vi "get_status.vi"(0 "connection ID in":refnum<k5>, 2 "command in":string, 3 "error in":errorcluster, 4 "设备编号":u8) -> (5 "connection ID out":refnum<k5>, 6 "Status received":string[](array[string]), 7 "error out":errorcluster)   [LabVIEW 2013]
panel:
  out "bytes written":i32
  out "Data Length":u16
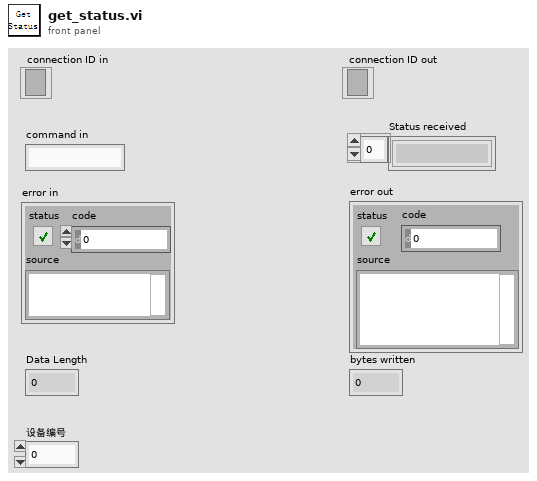
[diagram p1: front panel]
types:
  T1 = enum16{"Standard", "Buffered", "CRLF", "Immediate"}
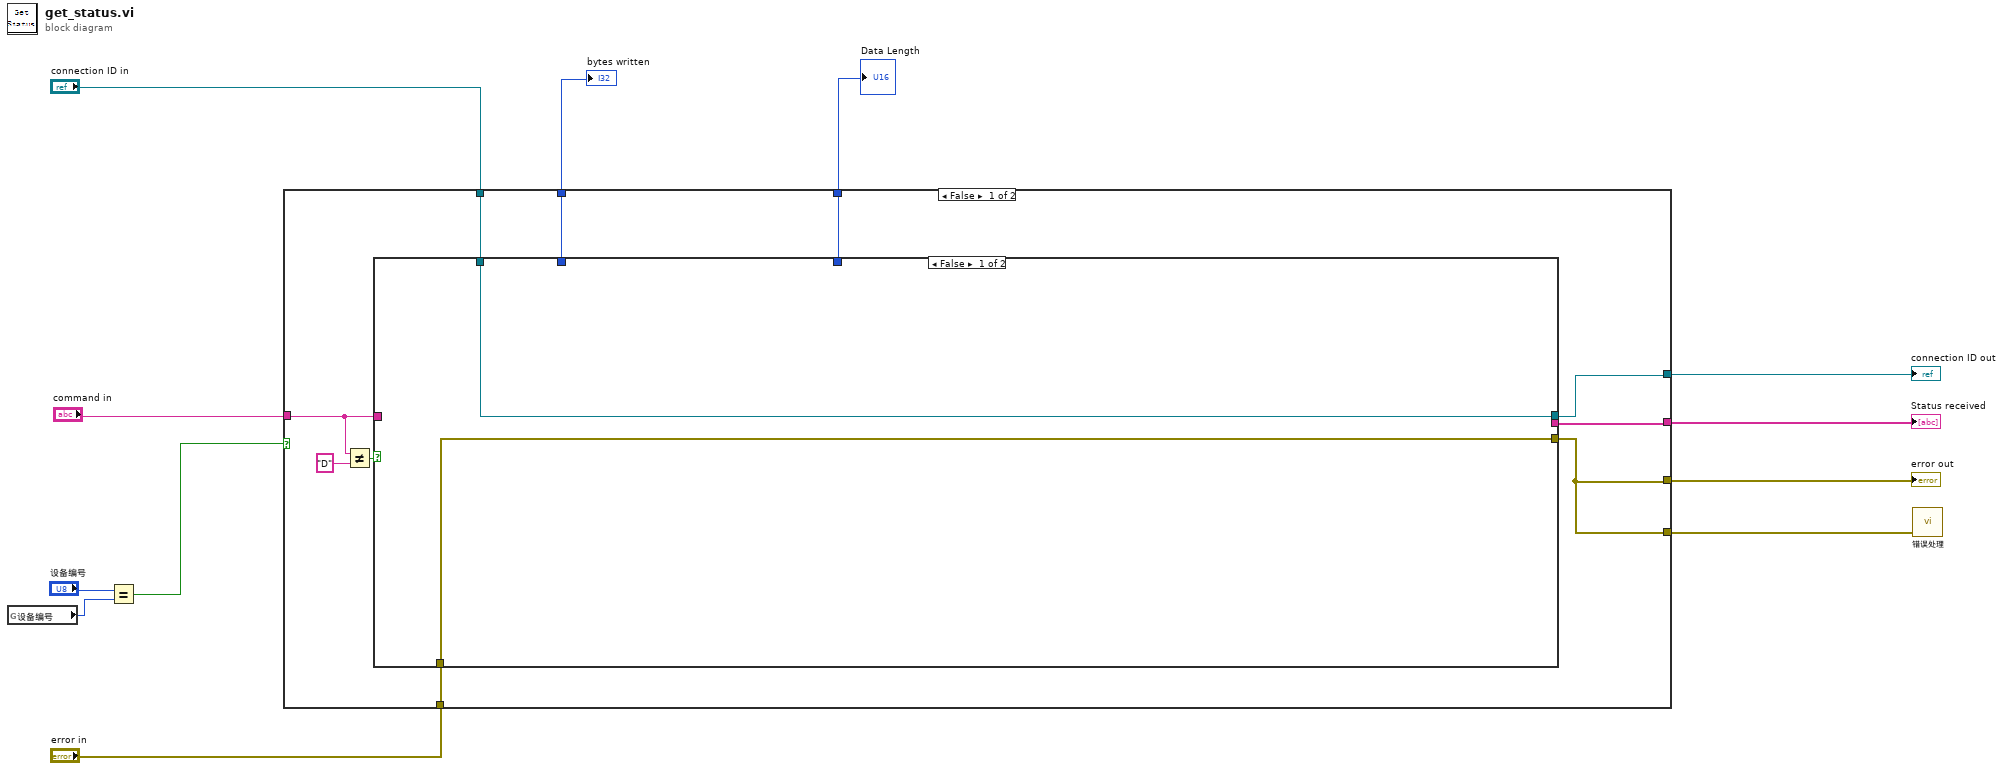
[diagram p0: block diagram]
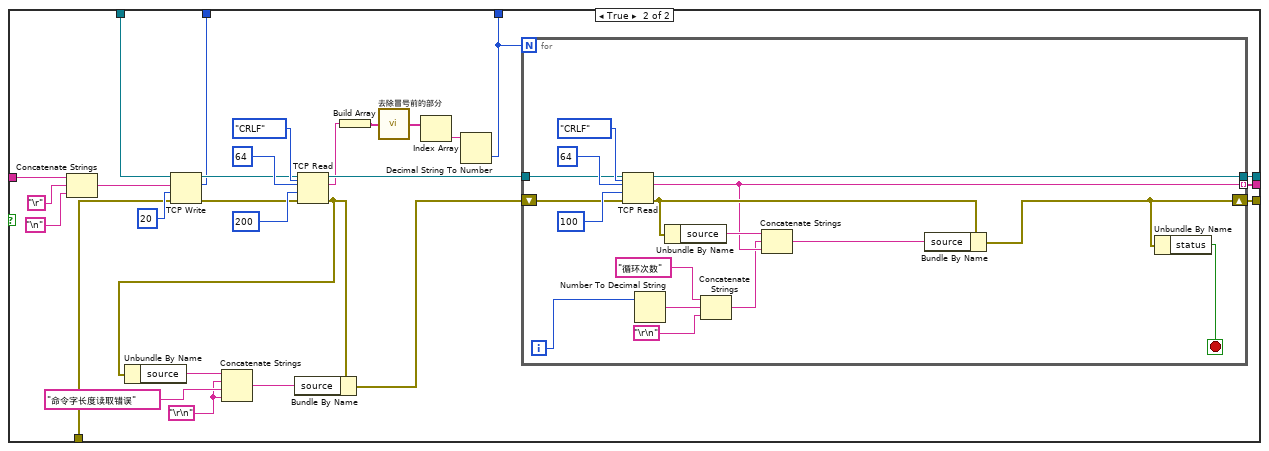
[diagram p2: hidden frame]
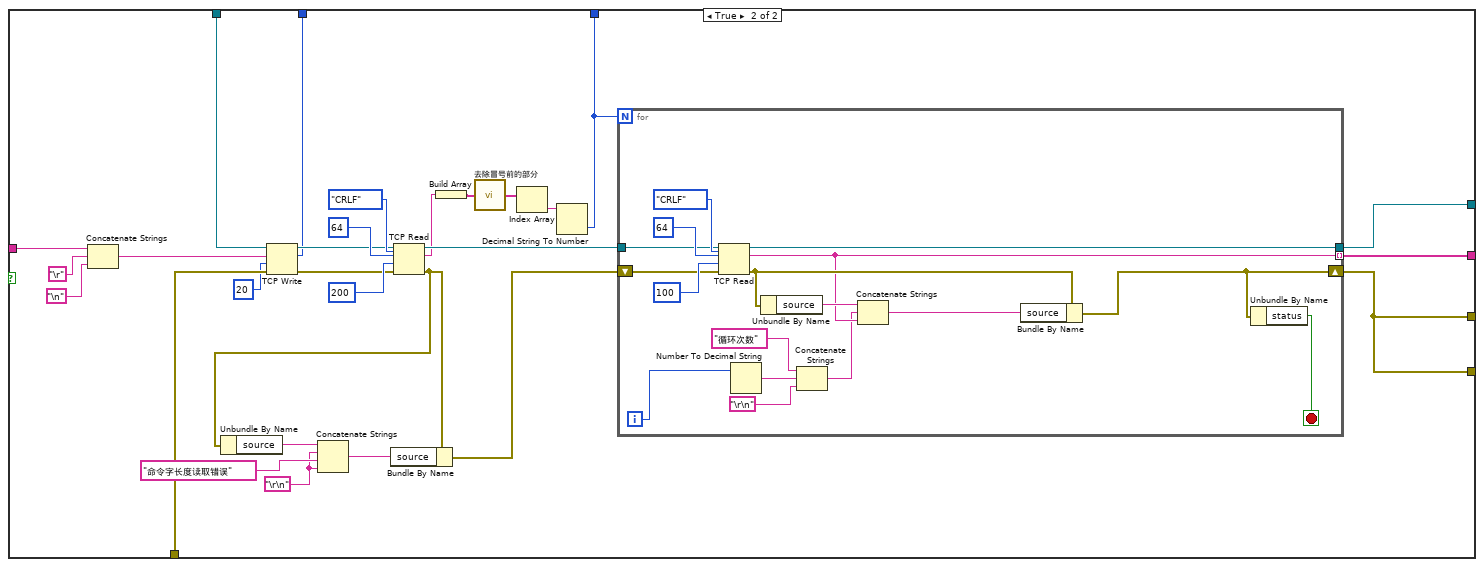
[diagram p3: hidden frame]
diagram:
  n1 = global read "设备编号.vi" "设备编号"() -> (w3:u8)
  n2 = Equal?(x="设备编号", y=w3) -> (x = y?=w2:bool)
  n3 = case shown="False" w2 {
    tunnel: [w21 w97] -> w12
    tunnel: [w22 w96] -> w11
    tunnel: "command in" -> [w13 w93]
    tunnel: "error in" -> [w17 w91]
    tunnel: [w18 w79] -> w8
    tunnel: [w19 w78] -> w7
    tunnel: [w16 w70] -> w6
    tunnel: "connection ID in" -> [w20 w71]
    tunnel: [w16 w70] -> w1
    frame False {
      n4 = Not Equal?(x=w13, y="D") -> (x != y?=w15:bool)
      n5 = case shown="False" w15 {
        tunnel: [w23 w32] -> w22
        tunnel: [_ w31] -> w21
        tunnel: w13 -> [_ w30]
        tunnel: w20 -> [w23 w29]
        tunnel: [_ w28] -> w19
        tunnel: [_ w27] -> w18
        tunnel: w17 -> [w24 w26]
        tunnel: [w24 w25] -> w16
        frame False {
        }
        frame True {
          w33 = "\r\n"
          n6 = Concatenate Strings(w30, "\r", "\n") -> (w50:string)
          n7 = TCP Write(connection ID=w29, data in=w50, error in (no error)=w26, 9:20 ("timeout ms (25000)")) -> (connection ID out=w45:refnum<k5>, bytes written=w28:i32, error out=w43:errorcluster)
          n8 = TCP Read(connection ID=w45, bytes to read=64, error in (no error)=w43, 7:T1."CRLF" ("mode (standard)"), 9:200 ("timeout ms (25000)")) -> (connection ID out=w44:refnum<k5>, data out=w42:string, error out=w36:errorcluster)
          n9 = Unbundle By Name(w36) -> ("source"=w34:string)
          n10 = Concatenate Strings(w34, w33, "命令字长度读取错误", w33) -> (w38:string)
          n11 = Bundle By Name(cluster=w36, "source"=w38) -> (w35:errorcluster)
          n12 = Build Array(w42) -> (w41:string[])
          n13 = call "去除冒号前的部分.vi"("返回值列表"=w41) -> ("返回值参数列表"=w40:string[])
          n14 = Index Array(array=w40) -> (element=w39:string)  [unwired: 1 in]
          n15 = Decimal String To Number(string=w39) -> (number=w27:i32)  [unwired: 2 in, 1 out]
          n16 = for {
            N: w27 -> [_]
            tunnel: [w66] -> w32
            tunnel: [w55] -> w31 mode=indexing
            shift-right: [w61] -> w25
            shift-left: w35 -> [w65]
            tunnel: w44 -> [w64]
            i -> [w58]
            stop <- w63 stop-if-true
            n17 = TCP Read(connection ID=w64, bytes to read=64, error in (no error)=w65, 7:T1."CRLF" ("mode (standard)"), 9:100 ("timeout ms (25000)")) -> (connection ID out=w66:refnum<k5>, data out=w55:string, error out=w62:errorcluster)
            n18 = Number To Decimal String(number=w58) -> (decimal integer string=w57:string)  [unwired: 1 in]
            n19 = Unbundle By Name(w62) -> ("source"=w60:string)
            n20 = Concatenate Strings("循环次数", w57, "\r\n") -> (w54:string)
            n21 = Concatenate Strings(w60, w54, w55) -> (w59:string)
            n22 = Bundle By Name(cluster=w62, "source"=w59) -> (w61:errorcluster)
            n23 = Unbundle By Name(w61) -> ("status"=w63:bool)
          }
        }
      }
    }
    frame True {
      w72 = "\r\n"
      n24 = Concatenate Strings(w93, "\r", "\n") -> (w92:string)
      n25 = TCP Write(connection ID=w71, data in=w92, error in (no error)=w91, 9:20 ("timeout ms (25000)")) -> (connection ID out=w86:refnum<k5>, bytes written=w78:i32, error out=w84:errorcluster)
      n26 = TCP Read(connection ID=w86, bytes to read=64, error in (no error)=w84, 7:T1."CRLF" ("mode (standard)"), 9:200 ("timeout ms (25000)")) -> (connection ID out=w85:refnum<k5>, data out=w83:string, error out=w75:errorcluster)
      n27 = Unbundle By Name(w75) -> ("source"=w73:string)
      n28 = Concatenate Strings(w73, w72, "命令字长度读取错误", w72) -> (w77:string)
      n29 = Bundle By Name(cluster=w75, "source"=w77) -> (w74:errorcluster)
      n30 = Build Array(w83) -> (w82:string[])
      n31 = call "去除冒号前的部分.vi"("返回值列表"=w82) -> ("返回值参数列表"=w81:string[])
      n32 = Index Array(array=w81) -> (element=w80:string)  [unwired: 1 in]
      n33 = Decimal String To Number(string=w80) -> (number=w79:i32)  [unwired: 2 in, 1 out]
      n34 = for {
        N: w79 -> [_]
        tunnel: [w111] -> w96
        tunnel: [w100] -> w97 mode=indexing
        shift-right: [w106] -> w70
        shift-left: w74 -> [w110]
        tunnel: w85 -> [w109]
        i -> [w103]
        stop <- w108 stop-if-true
        n35 = TCP Read(connection ID=w109, bytes to read=64, error in (no error)=w110, 7:T1."CRLF" ("mode (standard)"), 9:100 ("timeout ms (25000)")) -> (connection ID out=w111:refnum<k5>, data out=w100:string, error out=w107:errorcluster)
        n36 = Number To Decimal String(number=w103) -> (decimal integer string=w102:string)  [unwired: 1 in]
        n37 = Unbundle By Name(w107) -> ("source"=w105:string)
        n38 = Concatenate Strings("循环次数", w102, "\r\n") -> (w99:string)
        n39 = Concatenate Strings(w105, w99, w100) -> (w104:string)
        n40 = Bundle By Name(cluster=w107, "source"=w104) -> (w106:errorcluster)
        n41 = Unbundle By Name(w106) -> ("status"=w108:bool)
      }
    }
  }
  "connection ID out" <- w11
  "Status received" <- w12
  "error out" <- w6
  "Data Length" <- w8
  "bytes written" <- w7
  n42 = call "错误处理.vi"("error in (no error)"=w1) -> ()  [unwired: 2 in]
